vi "SWTrigEventReference.vi"() -> ()   [LabVIEW 2020]
uses:
  UDP_FGV.ctl
panel:
  in  "SWTRIGEventRef":refnum<event-registration>
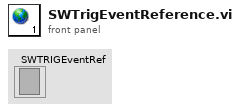
[diagram p1: front panel]
diagram:
